vi "APTopen.vi"(4 "error in (no error)":errorcluster) -> (0 "error out":errorcluster, 3 "reference out":refnum<k7>)   [LabVIEW 2013]
panel:
  in  "MG17Piezo":refnum<k7>(container)
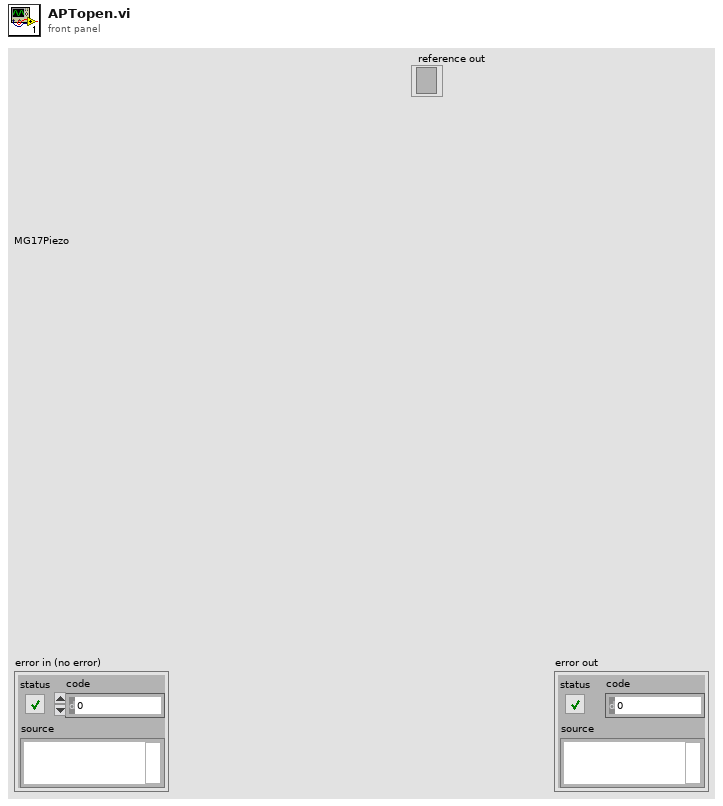
[diagram p1: front panel]
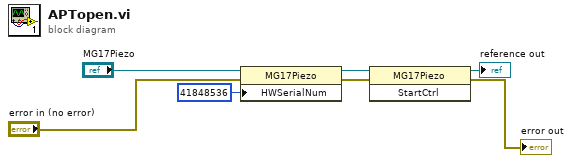
[diagram p0: block diagram]
diagram:
  n1 = property class="MG17Piezo"(reference="MG17Piezo", error in="error in (no error)", "HWSerialNum"=41848536) -> (reference out=w5:refnum<k7>, error out=w4:errorcluster)
  n2 = invoke class="MG17Piezo" method="StartCtrl"(reference=w5, error in=w4) -> (reference out=→"reference out":refnum<k7>, error out=→"error out":errorcluster)  [unwired: 1 in, 1 out]
